vi "setVariaControls.vi"(1 "LPFilterSetpointAngstrom":u16=6100, 2 "SWFilterSetpointAngstrom":u16=6000, 3 "NDFilterSetpointPercentx10":u16=500, 6 "error in (no error)":errorcluster, 9 "COMport":string="COM6") -> (0 "error out":errorcluster)   [LabVIEW 2015]
uses:
  superKSDK/05_Labview Driver/Examples/To ByteArray ([U16]).vi
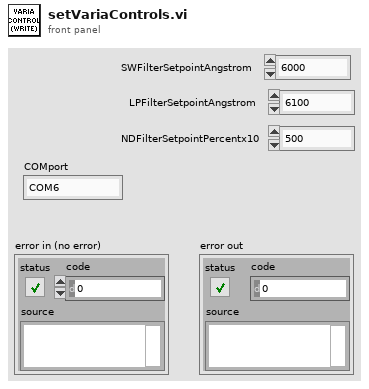
[diagram p1: front panel]
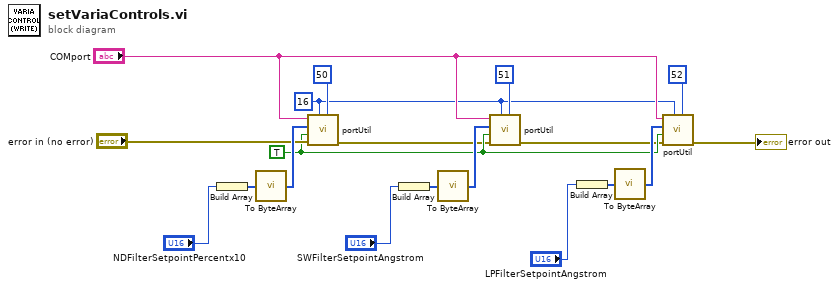
[diagram p0: block diagram]
diagram:
  w3 = TRUE ("WriteNotRead")
  w4 = u8 16 ("Destination")
  n1 = Build Array("NDFilterSetpointPercentx10") -> (w14:u16[])
  n2 = call-poly "To ByteArray.vi"("[U16]"=w14) -> ("PayloadByteArray"=w16:u8[])
  n3 = call "portUtil.vi"("Register"=u8 50, "Destination"=w4, "error in (no error)"="error in (no error)", "WriteNotRead"=w3, "Array"=w16, "COMport"="COMport") -> ("error out"=w2:errorcluster)  [unwired: 3 in, 2 out]
  n4 = Build Array("SWFilterSetpointAngstrom") -> (w7:u16[])
  n5 = call-poly "To ByteArray.vi"("[U16]"=w7) -> ("PayloadByteArray"=w8:u8[])
  n6 = call "portUtil.vi"("Register"=u8 51, "Destination"=w4, "error in (no error)"=w2, "WriteNotRead"=w3, "Array"=w8, "COMport"="COMport") -> ("error out"=w1:errorcluster)  [unwired: 3 in, 2 out]
  n7 = Build Array("LPFilterSetpointAngstrom") -> (w13:u16[])
  n8 = call-poly "To ByteArray.vi"("[U16]"=w13) -> ("PayloadByteArray"=w15:u8[])
  n9 = call "portUtil.vi"("Register"=u8 52, "Destination"=w4, "error in (no error)"=w1, "WriteNotRead"=w3, "Array"=w15, "COMport"="COMport") -> ("error out"=→"error out":errorcluster)  [unwired: 3 in, 2 out]
